vi "4Pi AA Find Crossing.vi"(0 "Fit Parameters 01":dbl[](array[numeric]), 11 "Fit Parameters 02":dbl[](array[numeric])) -> (8 "X Crossing Position":dbl)   [LabVIEW 2020]
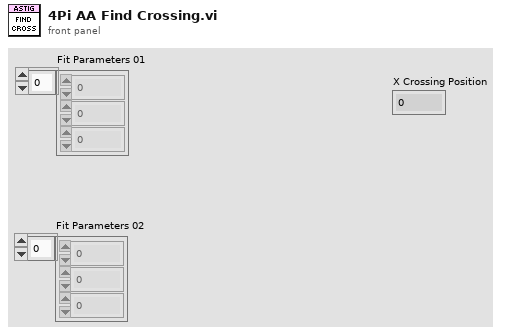
[diagram p1: front panel]
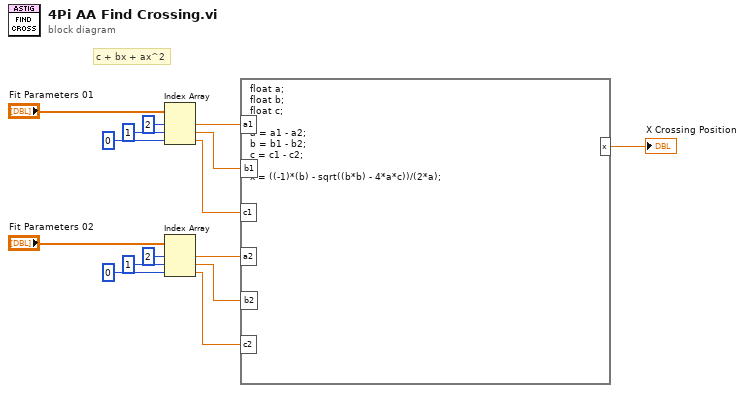
[diagram p0: block diagram]
diagram:
  # "c + bx + ax^2"
  n1 = Index Array(array="Fit Parameters 01", index #1=2 ("index"), index #2=1 ("index"), index #3=0 ("index")) -> (element #1=w7:dbl, element #2=w3:dbl, element #3=w5:dbl)
  n2 = Index Array(array="Fit Parameters 02", index #1=2 ("index"), index #2=1 ("index"), index #3=0 ("index")) -> (element #1=w6:dbl, element #2=w2:dbl, element #3=w4:dbl)
  n3 = formula code="float a;\nfloat b;\nfloat c;\n\na = a1 - a2;\nb = b1 - b2;\nc = c1 - c2;\n\nx = ((-1)*(b) - sqrt((b*b) - 4*a*c))/(2*a);"("a1"=w7, "b1"=w3, "c1"=w5, "a2"=w6, "b2"=w2, "c2"=w4) -> ("x"=→"X Crossing Position":dbl)
